vi "EventGenerator.vi"(6 "Dist Para Toque":dbl=130.0, 8 "Tol para ang posse":dbl=0.3, 9 "Dist Para posse":dbl=180.0, 10 "IA State Input":T1, 11 "lado, readius, stretch":i32[](array[numeric])) -> (2 "IA State Output":T1)   [LabVIEW 2017]
uses:
  AI Input.ctl
  AI Robot.ctl
  Intel/Functions Enum.ctl
  Intel/AttackerStates.ctl
  Path Planning/RRT/PathDests.ctl
  Path Planning/RRT/PathDest.ctl
  AI Ball.ctl
  Field Size.ctl
  AI Judge.ctl
  Intel/Command Enum.ctl
  Util/Events/Events.ctl
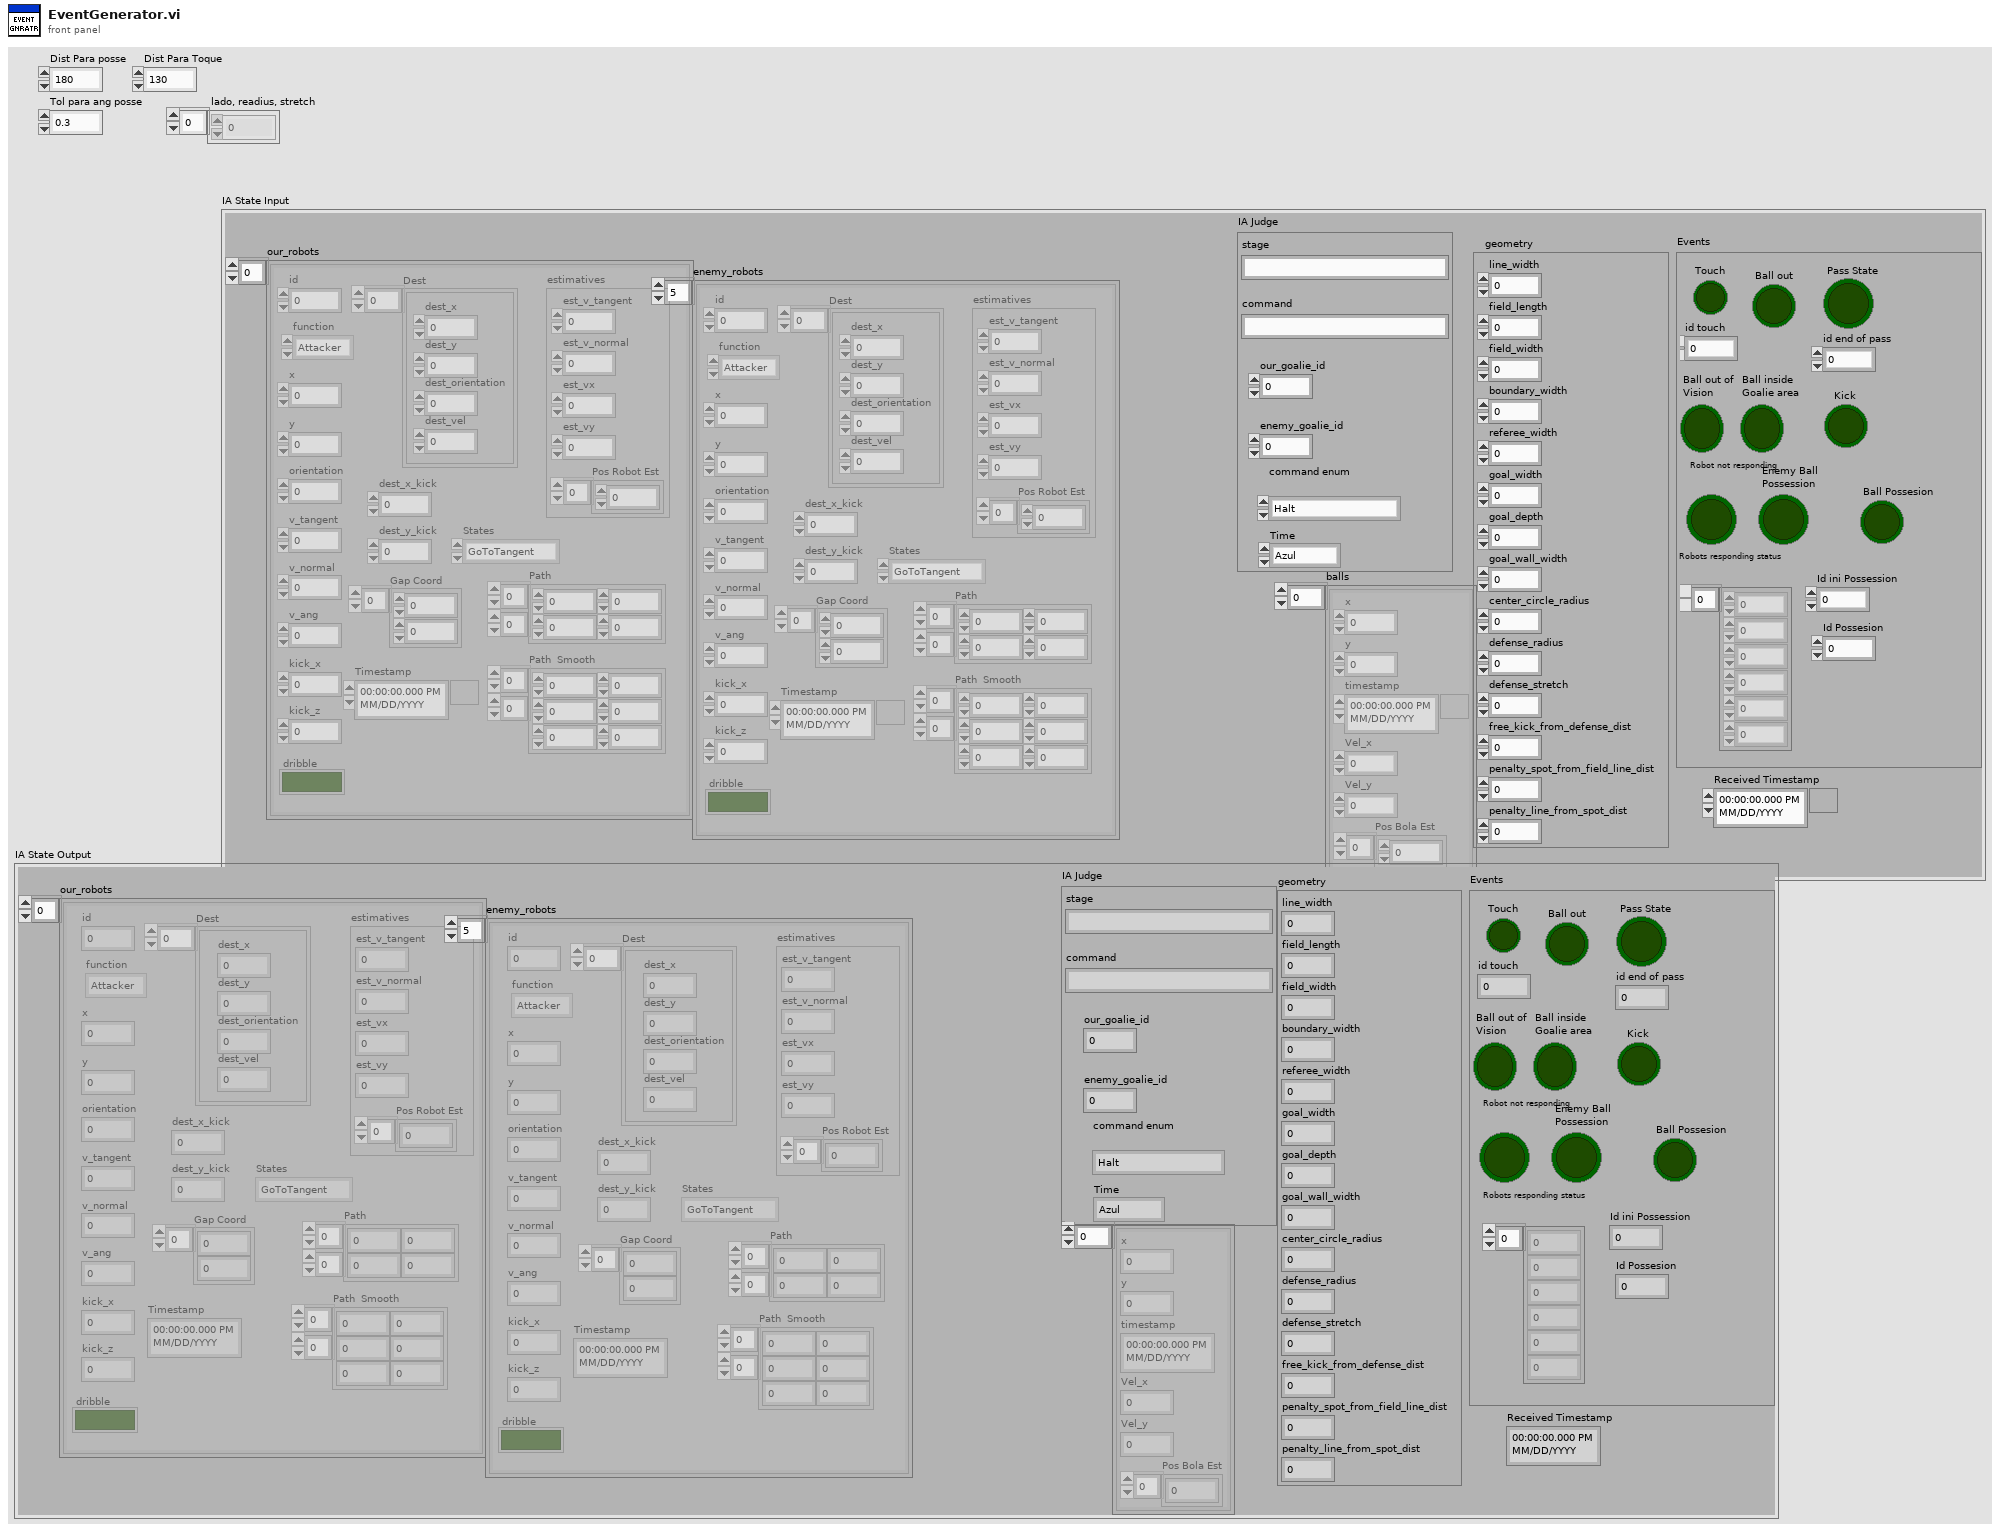
[diagram p1: front panel]
types:
  T1 = typedef "AI Input.ctl" = cluster{"our_robots":T2[], "enemy_robots":T2[], "balls":T7[], "geometry":T8, "IA Judge":T9, "Received Timestamp":timestamp, "Events":T11}
  T2 = typedef "AI Robot.ctl" = cluster{"id":u32, "function":T3, "x":dbl, "y":dbl, "orientation":dbl, "v_tangent":dbl, "v_normal":dbl, "v_ang":dbl, "kick_x":dbl, "kick_z":dbl, "dribble":bool, "Timestamp":timestamp, "estimatives":cluster{"est_v_tangent":dbl, "est_v_normal":dbl, "est_vx":dbl, "est_vy":dbl, "Pos Robot Est":dbl[]}, "dest_x_kick":dbl, "dest_y_kick":dbl, "Gap Coord":dbl[], "States":T4, "Path ":dbl[][], "Path  Smooth":dbl[][], "Dest":T5}
  T3 = typedef "Functions Enum.ctl" = enum16{"Attacker", "Goalie", "Defender", "Striker", "Goto 0", "Dummy", "Kicker", "ZigZag"}
  T4 = typedef "AttackerStates.ctl" = enum16{"Pass", "GoToTangent", "BallGetting", "GoToKick", ""}
  T5 = typedef "PathDests.ctl" = T6[]
  T6 = typedef "PathDest.ctl" = cluster{"dest_x":dbl, "dest_y":dbl, "dest_orientation":dbl, "dest_vel":dbl}
  T7 = typedef "AI Ball.ctl" = cluster{"x":dbl, "y":dbl, "timestamp":timestamp, "Vel_x":dbl, "Vel_y":dbl, "Pos Bola Est":dbl[]}
  T8 = typedef "Field Size.ctl" = cluster{"line_width":u32, "field_length":u32, "field_width":u32, "boundary_width":u32, "referee_width":u32, "goal_width":u32, "goal_depth":u32, "goal_wall_width":u32, "center_circle_radius":u32, "defense_radius":u32, "defense_stretch":u32, "free_kick_from_defense_dist":u32, "penalty_spot_from_field_line_dist":u32, "penalty_line_from_spot_dist":u32}
  T9 = typedef "AI Judge.ctl" = cluster{"stage":string, "command":string, "our_goalie_id":dbl, "enemy_goalie_id":dbl, "command enum":T10, "Time":enum16{"Azul", "Amarelo"}}
  T10 = typedef "Command Enum.ctl" = enum16{"Halt", "Stop", "Force Start", "PKA Normal Start", "Prepare Kickoff Ally", "PKE Normal Start", "Prepare Kickoff Enemy", "Prepare Penalty Ally", "PPA Normal Start", "Prepare Penalty Enemy", "PPE Normal Start", "Direct Free Enemy", "Direct Free Ally", "Indirect Free Enemy", "Indirect Free Ally", "Timeout Enemy", "Timeout Ally", "Goal Enemy", "Goal Ally", "Ball Placement Enemy", "Ball Placement Ally", "Normal Half Time", "Extra Time Break", "Extra Half Time", "None", "Post Game"}
  T11 = typedef "Events.ctl" = cluster{"Touch":bool, "Ball out":bool, "id touch":dbl, "Ball out of \nVision":bool, "Ball inside \nGoalie area":bool, "Robot not responding":bool, "Robots responding status":dbl[], "Enemy Ball \nPossession":bool, "Pass State":bool, "id end of pass":dbl, "Kick":bool, "Id ini Possession":dbl, "Ball Possesion":bool, "Id Possesion":dbl}
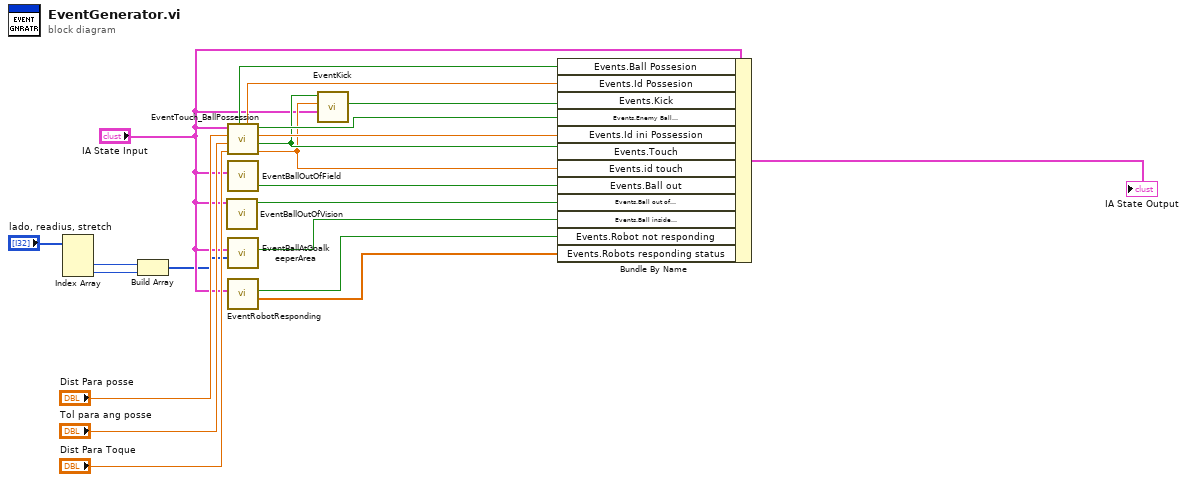
[diagram p0: block diagram]
diagram:
  n1 = Index Array(array="lado, readius, stretch") -> (element #2=w15:i32, element #3=w14:i32)  [unwired: 3 in, 1 out]
  n2 = Build Array(w15, w14) -> (w1:i32[])
  n3 = call "EventBallOutOfVision.vi"("IA State"="IA State Input") -> ("Bola fora da Visão?"=w20:bool)  [unwired: 10 in]
  n4 = call "EventTouch_BallPossession.vi"("Dist Para Toque"="Dist Para Toque", "Tol para ang posse"="Tol para ang posse", "Dist Para posse"="Dist Para posse", "IA State"="IA State Input") -> ("id touch"=w8:dbl, "Toque"=w9:bool, "id ini possesion"=w10:dbl, "Posse inimigo"=w11:bool, "id possesion"=w3:dbl, "Posse nossa"=w4:bool)  [unwired: 2 in]
  n5 = call "EventBallOutOfField.vi"("IA State"="IA State Input") -> ("Bola fora do campo?"=w21:bool)  [unwired: 10 in]
  n6 = call "EventBallAtGoalkeeperArea.vi"("Field defense"=w1, "IA State"="IA State Input") -> ("Ball at goalkeeper area ?"=w19:bool)  [unwired: 9 in]
  n7 = call "EventRobotResponding.vi"("IA State 2"="IA State Input") -> ("Robot responding status"=w17:dbl[], "Is there a robot not responding?"=w18:bool)  [unwired: 8 in]
  n8 = call "EventKick.vi"("Toque"=w9, "id"=w8, "IA State Input"="IA State Input") -> ("Kick"=w12:bool)  [unwired: 7 in]
  n9 = Bundle By Name(cluster="IA State Input", "Events.Ball Possesion"=w4, "Events.Id Possesion"=w3, "Events.Kick"=w12, "Events.Enemy Ball \nPossession"=w11, "Events.Id ini Possession"=w10, "Events.Touch"=w9, "Events.id touch"=w8, "Events.Ball out"=w21, "Events.Ball out of \nVision"=w20, "Events.Ball inside \nGoalie area"=w19, "Events.Robot not responding"=w18, "Events.Robots responding status"=w17) -> (→"IA State Output":T1)
